vi "Write belongsTo.vi"(8 "error in (no error)":errorcluster, 10 "belongsTo":string, 11 "FSM.Port in":refnum<class "FSM.Port.lvclass">) -> (0 "error out":errorcluster, 3 "FSM.Port out":refnum<class "FSM.Port.lvclass">)   [LabVIEW 2020, in "FSM.Port.lvclass"]
uses:
  FSM.Port.lvclass
  FSM.Port.lvclass/FSM.Port.ctl
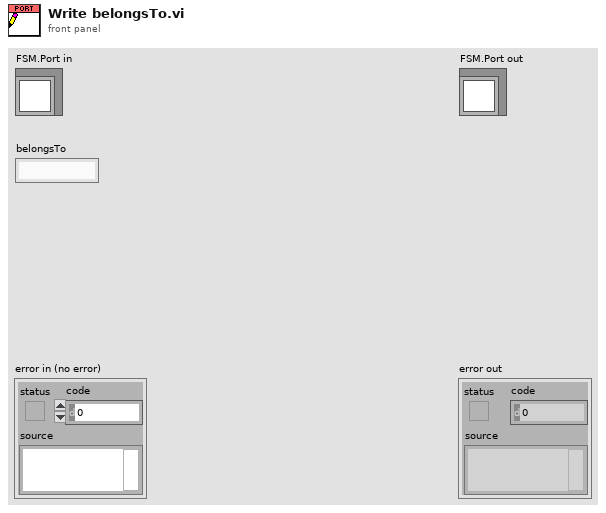
[diagram p1: front panel]
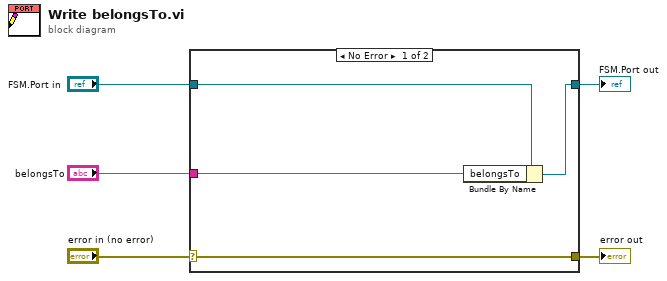
[diagram p0: block diagram]
diagram:
  n1 = case shown="No Error" "error in (no error)" {
    selector: "error in (no error)" -> [w9 w10]
    tunnel: [w9 w10] -> w4
    tunnel: [w7 w11] -> w2
    tunnel: "FSM.Port in" -> [w8 w11]
    tunnel: "belongsTo" -> [w6 _]
    frame No Error {
      n2 = Bundle By Name(cluster=w8, "belongsTo"=w6) -> (w7:refnum<class "FSM.Port.lvclass">)
    }
    frame Error {
    }
  }
  "error out" <- w4
  "FSM.Port out" <- w2
